vi "RFID Open.vi"() -> ()   [LabVIEW 2018]
uses:
  <vilib>/Instr/_visa.llb/VISA Configure Serial Port (Instr).vi
panel:
  out "received":string
  in  "ComPort":refnum<visa-resource-name>="COM10"
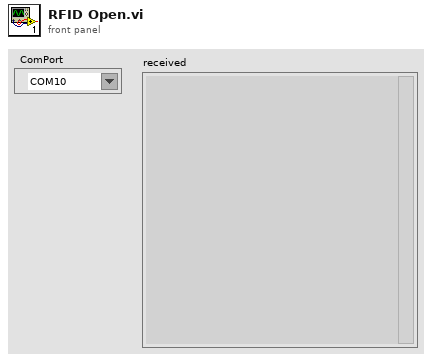
[diagram p1: front panel]
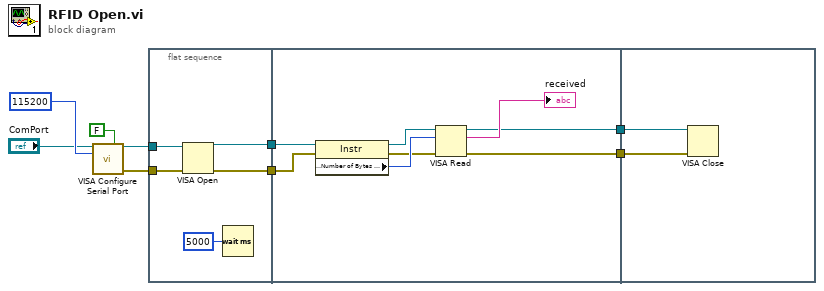
[diagram p0: block diagram]
diagram:
  n1 = call-poly "VISA Configure Serial Port"("VISA resource name"="ComPort", "Enable Termination\nChar (T)"=FALSE ("Enable Termination\nChar (T)"), "baud rate (9600)"=u32 115200 ("Serial Settings:Baud Rate")) -> ("VISA resource name out"=w5:refnum<visa-resource-name>, "error out"=w6:errorcluster)  [unwired: 11 in]
  n2 = flat-sequence {
    tunnel: w6 -> [w14]
    tunnel: w5 -> [w13]
    tunnel: [w11] -> w4
    tunnel: [w10] -> w3
    tunnel: w4 -> [w19]
    tunnel: w3 -> [w18]
    tunnel: [w16] -> w2
    tunnel: [w15] -> w1
    tunnel: w2 -> [w24]
    tunnel: w1 -> [w23]
    frame #0 {
      n3 = VISA Open(error in (no error)=w14, VISA resource name=w13) -> (VISA resource name=w11:refnum<visa-resource-name>, error out=w10:errorcluster)  [unwired: 3 in]
      n4 = Wait (ms)(milliseconds to wait=u32 5000) -> ()  [unwired: 1 out]
    }
    frame #1 {
      n5 = property class="Instr"(reference=w19, error in=w18) -> (reference out=w21:refnum<visa-resource-name>, error out=w20:errorcluster, "Serial Settings:Number of Bytes at Serial Port"=w22:u32)
      n6 = VISA Read(VISA resource name=w21, byte count=w22, error in (no error)=w20) -> (VISA resource name out=w16:refnum<visa-resource-name>, read buffer=→"received":string, error out=w15:errorcluster)  [unwired: 1 out]
    }
    frame #2 {
      n7 = VISA Close(VISA resource name=w24, error in (no error)=w23) -> ()  [unwired: 1 out]
    }
  }
